vi "get waveform.vi"(8 "error in (no error)":errorcluster caption="에러 입력(에러 없음)", 11 "Text File 입력":refnum<class "Text File.lvclass">) -> (0 "error out":errorcluster caption="에러 출력", 2 "waveform":waveform(dbl), 3 "Text File 출력":refnum<class "Text File.lvclass">)   [LabVIEW 2020, in "Text File.lvclass"]
uses:
  Text File.lvclass
  Text File.lvclass/Text File.ctl
  Waveform Obj/Waveform Obj.lvclass/Waveform Obj.ctl
  Accessors/Read Text_Sampling Rate.vi
  Accessors/Read Data.vi
  Waveform Obj/Accessors/Read sampling rate.vi
  <vilib>/measure/maresamp.llb/Resample Waveform (single shot).vi
  <vilib>/measure/NI_MAPro.lvlib
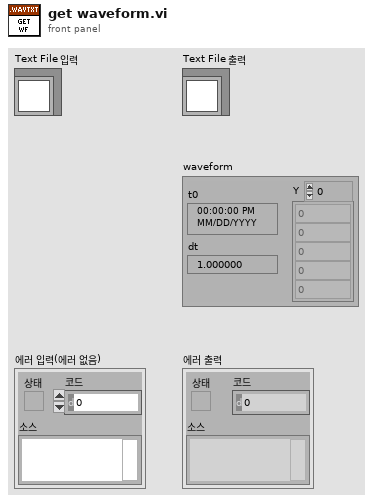
[diagram p1: front panel]
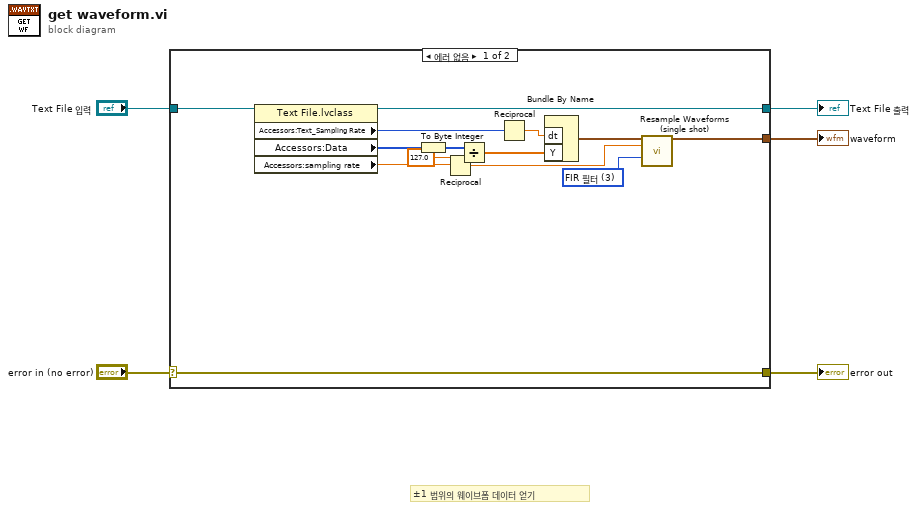
[diagram p0: block diagram]
diagram:
  # "±1 범위의 웨이브폼 데이터 얻기"
  n1 = case shown="에러 없음" "error in (no error)" {
    selector: "error in (no error)" -> [w19 w21]
    tunnel: [w19 w21] -> w5
    tunnel: [w17 w20] -> w4
    tunnel: "Text File 입력" -> [w18 w20]
    tunnel: [w9 _] -> w1
    frame No Error {
      w6 = u16 3 items=["강제 변환", "선형", "스플라인", "FIR 필터"] ("interpolation mode")
      n2 = property class="Text File.lvclass"(reference=w18) -> (reference out=w17:refnum<class "Text File.lvclass">, "Accessors:Text_Sampling Rate"=w10:i32, "Accessors:Data"=w15:u16[], "Accessors:sampling rate"=w7:dbl)  [unwired: 1 in, 1 out]
      n3 = To Byte Integer(number=w15) -> (8bit integer=w14:i8[])
      n4 = Reciprocal(x=w7) -> (1/x=w8:dbl)
      n5 = Divide(x=w14, y=127.0) -> (x/y=w13:dbl[])
      n6 = Reciprocal(x=w10) -> (1/x=w12:dbl)
      n7 = Bundle By Name("dt"=w12, "Y"=w13) -> (w11:waveform(dbl))  [unwired: 1 in]
      n8 = call-poly <vilib>:"Resample Waveforms (single shot).vi"("waveform in"=w11, "dt"=w8, "interpolation mode"=w6) -> ("resampled waveform out"=w9:waveform(dbl))  [unwired: 9 in, 3 out]
    }
    frame Error {
    }
  }
  "error out" <- w5
  "Text File 출력" <- w4
  "waveform" <- w1
